vi "Forward.vi"(8 "error in (no error)":errorcluster, 10 "how close":dbl) -> (0 "error out":errorcluster, 2 "Done":bool)   [LabVIEW 2019]
uses:
  Simulated Robot/Simulation SubVIs/Simulation SubVIs.lvlib
panel:
  out "Diff. x Z":dbl
  out "Right sonar":dbl
  out "Left sonar":dbl
  out "Right":dbl
  out "Left":dbl
  out "Diff.":dbl
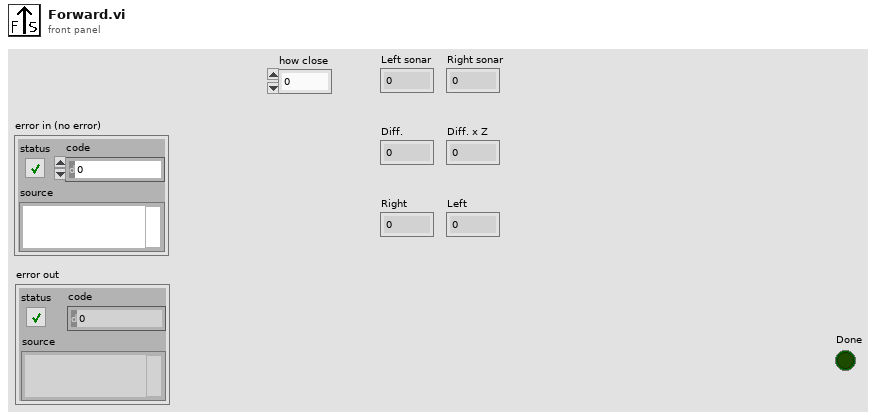
[diagram p1: front panel]
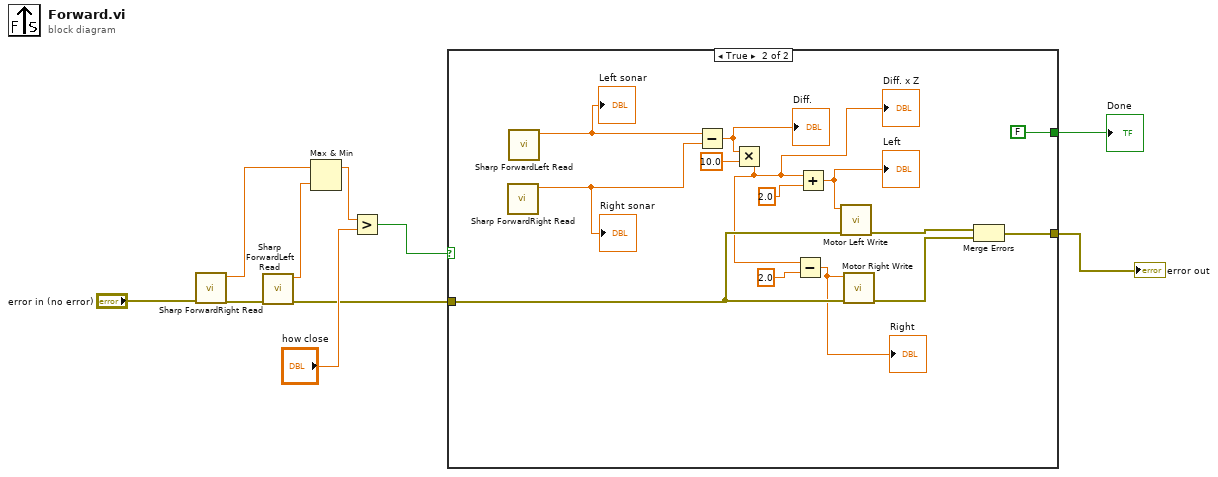
[diagram p0: block diagram]
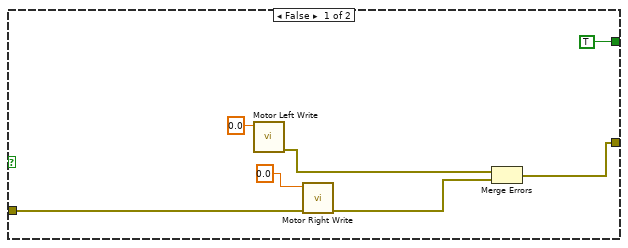
[diagram p2: hidden frame]
diagram:
  n1 = call "Sharp ForwardRight Read.vi"("error in (no error)"="error in (no error)") -> ("error out"=w5:errorcluster, "ForwardRight Distance (m)"=w2:dbl)  [unwired: 9 in]
  n2 = call "Sharp ForwardLeft Read.vi"("error in (no error)"=w5) -> ("error out"=w6:errorcluster, "ForwardLeft Distance (m)"=w3:dbl)  [unwired: 9 in]
  n3 = Max & Min(x=w2, y=w3) -> (max(x,y)=w1:dbl)  [unwired: 1 out]
  n4 = Greater?(x=w1, y="how close") -> (0:w8:bool)
  n5 = case shown="True" w8 {
    tunnel: [w13 w29] -> w10
    tunnel: w6 -> [w12 w28]
    tunnel: [TRUE ("Done") FALSE ("Done")] -> w7
    frame False {
      n6 = call "Motor Left Write.vi"("left motor ccw velocity (rad/s)"=0.0) -> ("error out"=w17:errorcluster)  [unwired: 10 in]
      n7 = call "Motor Right Write.vi"("error in (no error)"=w12, "right motor ccw velocity (rad/s)"=0.0) -> ("error out"=w16:errorcluster)  [unwired: 9 in]
      n8 = Merge Errors(w17, w16) -> (w13:errorcluster)
    }
    frame True {
      n9 = call "Sharp ForwardRight Read.vi"() -> ("ForwardRight Distance (m)"=w20:dbl)  [unwired: 10 in, 1 out]
      "Right sonar" <- w20
      n10 = call "Sharp ForwardLeft Read.vi"() -> ("ForwardLeft Distance (m)"=w21:dbl)  [unwired: 10 in, 1 out]
      "Left sonar" <- w21
      n11 = Subtract(x=w21, y=w20) -> (x-y=w27:dbl)
      "Diff." <- w27
      n12 = Multiply(x=w27, y=10.0) -> (x*y=w19:dbl)
      "Diff. x Z" <- w19
      n13 = Subtract(x=w19, y=2.0) -> (x-y=w24:dbl)
      "Right" <- w24
      n14 = Add(x=w19, y=2.0 ("left motor ccw velocity (rad/s)")) -> (x+y=w23:dbl)
      "Left" <- w23
      n15 = call "Motor Left Write.vi"("error in (no error)"=w28, "left motor ccw velocity (rad/s)"=w23) -> ("error out"=w30:errorcluster)  [unwired: 9 in]
      n16 = call "Motor Right Write.vi"("error in (no error)"=w28, "right motor ccw velocity (rad/s)"=w24) -> ("error out"=w31:errorcluster)  [unwired: 9 in]
      n17 = Merge Errors(w30, w31) -> (w29:errorcluster)
    }
  }
  "error out" <- w10
  "Done" <- w7
